vi "GetExternalInterfaceString.vi"(8 "ErrorIn":errorcluster, 11 "ReferenceIn":refnum<class "AppConfigJSON.lvclass">) -> (0 "ErrorOut":errorcluster, 1 "String":string, 2 "Identification":string, 3 "ReferenceOut":refnum<class "AppConfigJSON.lvclass">)   [LabVIEW 2021, in "AppConfigJSON.lvclass"]
uses:
  AppConfigJSON.lvclass
  <vilib>/JDP Science/JSONtext/Config Files/Config File.lvclass
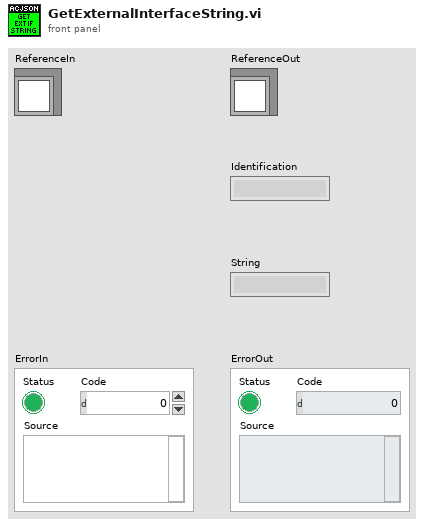
[diagram p1: front panel]
types:
  T1 = typedef "AppConfigJSON.lvclass/ObjectAttributes.ctl" = cluster{"Name":string, "ConfigFilePath":path, "Objects":T2[], "ApplicationBasePath":path, "ObjectName":string}
  T2 = typedef "IApplicationConfiguration.lvclass/ObjectDataDetails.ctl" = cluster{"ObjectName":string, "ObjectType":string, "Interfaces":T3[]}
  T3 = typedef "IApplicationConfiguration.lvclass/ObjectData.ctl" = cluster{"Label":string, "ObjectName":string, "Type":string}
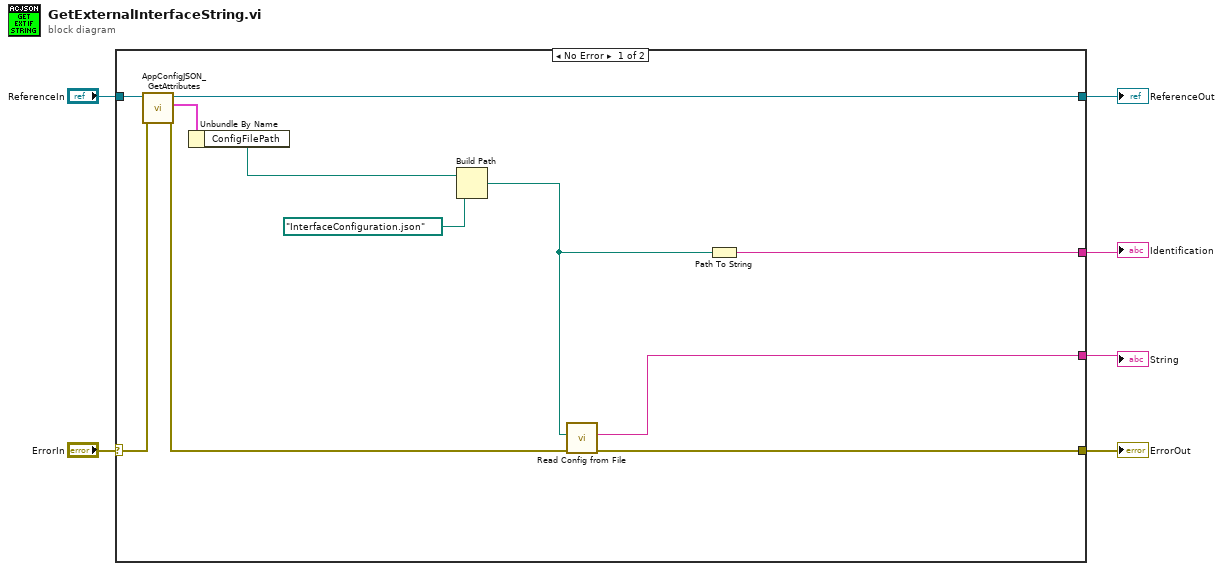
[diagram p0: block diagram]
diagram:
  n1 = case shown="No Error" "ErrorIn" {
    selector: "ErrorIn" -> [w16 w18]
    tunnel: [w15 w18] -> w5
    tunnel: [w12 w17] -> w3
    tunnel: "ReferenceIn" -> [w13 w17]
    tunnel: [w11 _] -> w2
    tunnel: [w10 _] -> w1
    frame No Error {
      n2 = call "AppConfigJSON_GetAttributes.vi"("ErrorIn"=w16, "ReferenceIn"=w13) -> ("ErrorOut"=w15:errorcluster, "Data"=w14:T1, "ReferenceOut"=w12:refnum<class "AppConfigJSON.lvclass">)  [unwired: 6 in, 1 out]
      n3 = Unbundle By Name(w14) -> ("ConfigFilePath"=w8:path)
      n4 = Build Path(base path=w8, name or relative path=path "InterfaceConfiguration.json") -> (appended path=w7:path)
      n5 = call <vilib>:"Read Config from File.vi"("error in (no error)"=w15, "config file path"=w7) -> ("<JSON>Config"=w11:string)  [unwired: 6 in, 3 out]
      n6 = Path To String(path=w7) -> (string=w10:string)
    }
    frame Error {
    }
  }
  "ErrorOut" <- w5
  "ReferenceOut" <- w3
  "String" <- w2
  "Identification" <- w1
